vi "Measure Calibration Data.vi"(5 "Standard (0: Open)":u16(ring) items=["Open", "Short", "Load", "Through", "Isolation", "Gain Phase Open", "Gain Phase Short", "Gain Phase Load", "Gain Phase Through", "Gain Phase Isolation"], 7 "Channel (1)":i32=1, 8 "error in (no error)":errorcluster, 9 "Port 2 - stimulus (2)":i32=2, 10 "Port 1 - response (1)":i32=1, 11 "VISA resource name":refnum<visa-resource-name>) -> (0 "error out":errorcluster, 3 "VISA resource name out":refnum<visa-resource-name>)   [LabVIEW 2020, in "Agilent ENA Series.lvlib"]
doc: "Measures the calibration data, for selected channel, of the open, short, load, through standard or isolation of the specified ports."
uses:
  <instrlib>/Agilent ENA Series/Agilent ENA Series.lvlib
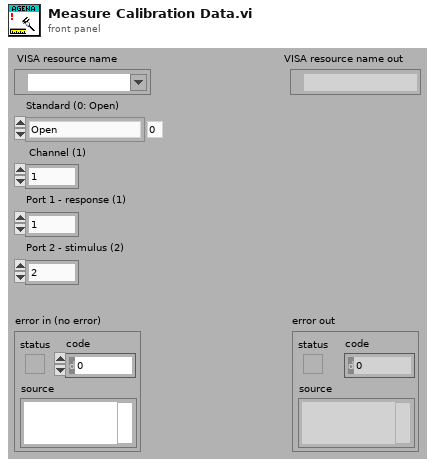
[diagram p1: front panel]
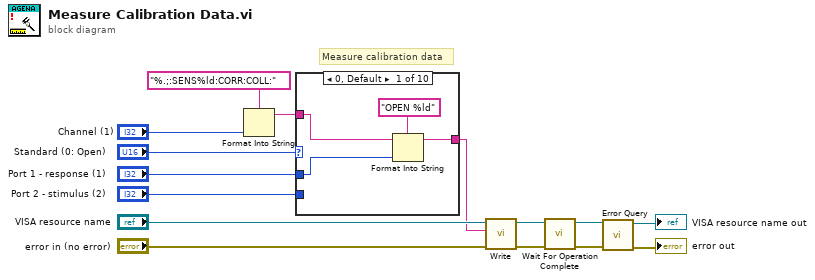
[diagram p0: block diagram]
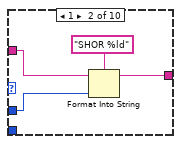
[diagram p2: hidden frame]
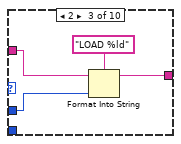
[diagram p3: hidden frame]
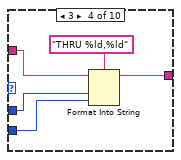
[diagram p4: hidden frame]
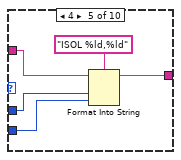
[diagram p5: hidden frame]
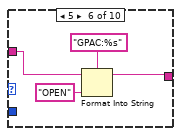
[diagram p6: hidden frame]
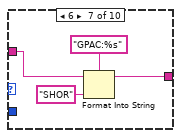
[diagram p7: hidden frame]
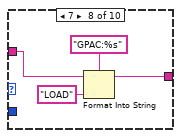
[diagram p8: hidden frame]
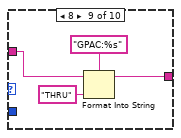
[diagram p9: hidden frame]
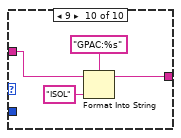
[diagram p10: hidden frame]
diagram:
  # "Measure calibration data"
  n1 = Format Into String(format string="%.;:SENS%ld:CORR:COLL:", "Channel (1)") -> (resulting string=w8:string)  [unwired: 2 in, 1 out]
  n2 = case shown="0, Default" "Standard (0: Open)" {
    tunnel: "Port 1 - response (1)" -> [w17 w21 w25 w30 w35 _ _ _ _ _]
    tunnel: "Port 2 - stimulus (2)" -> [_ _ _ w28 w33 _ _ _ _ _]
    tunnel: w8 -> [w18 w22 w26 w31 w36 w40 w43 w47 w51 w55]
    tunnel: [w16 w20 w24 w29 w34 w38 w42 w46 w50 w54] -> w7
    frame 0, Default {
      n3 = Format Into String(format string="OPEN %ld", initial string=w18, w17) -> (resulting string=w16:string)  [unwired: 1 in, 1 out]
    }
    frame 1 {
      n4 = Format Into String(format string="SHOR %ld", initial string=w22, w21) -> (resulting string=w20:string)  [unwired: 1 in, 1 out]
    }
    frame 2 {
      n5 = Format Into String(format string="LOAD %ld", initial string=w26, w25) -> (resulting string=w24:string)  [unwired: 1 in, 1 out]
    }
    frame 3 {
      n6 = Format Into String(format string="THRU %ld,%ld", initial string=w31, w30, w28) -> (resulting string=w29:string)  [unwired: 1 in, 1 out]
    }
    frame 4 {
      n7 = Format Into String(format string="ISOL %ld,%ld", initial string=w36, w35, w33) -> (resulting string=w34:string)  [unwired: 1 in, 1 out]
    }
    frame 5 {
      n8 = Format Into String(format string="GPAC:%s", initial string=w40, "OPEN" ("input 1")) -> (resulting string=w38:string)  [unwired: 1 in, 1 out]
    }
    frame 6 {
      n9 = Format Into String(format string="GPAC:%s", initial string=w43, "SHOR" ("input 1")) -> (resulting string=w42:string)  [unwired: 1 in, 1 out]
    }
    frame 7 {
      n10 = Format Into String(format string="GPAC:%s", initial string=w47, "LOAD" ("input 1")) -> (resulting string=w46:string)  [unwired: 1 in, 1 out]
    }
    frame 8 {
      n11 = Format Into String(format string="GPAC:%s", initial string=w51, "THRU" ("input 1")) -> (resulting string=w50:string)  [unwired: 1 in, 1 out]
    }
    frame 9 {
      n12 = Format Into String(format string="GPAC:%s", initial string=w55, "ISOL" ("input 1")) -> (resulting string=w54:string)  [unwired: 1 in, 1 out]
    }
  }
  n13 = call <instrlib>:"Write.vi"("error in (no error)"="error in (no error)", "String ()"=w7, "VISA resource name"="VISA resource name") -> ("error out"=w3:errorcluster, "VISA resource name out"=w4:refnum<visa-resource-name>)  [unwired: 6 in, 1 out]
  n14 = call <instrlib>:"Wait For Operation Complete.vi"("error in (no error)"=w3, "VISA resource name"=w4) -> ("error out"=w1:errorcluster, "VISA resource name out"=w2:refnum<visa-resource-name>)  [unwired: 8 in]
  n15 = call <instrlib>:"Error Query.vi"("error in (no error)"=w1, "VISA resource name"=w2) -> ("error out"=→"error out":errorcluster, "VISA resource name out"=→"VISA resource name out":refnum<visa-resource-name>)  [unwired: 6 in, 2 out]
